vi "program_supply_arduino.vi"() -> ()   [LabVIEW 2018]
uses:
  <vilib>/MakerHub/LINX/Public/Peripherals/Analog/Analog Read 1 Chan.vi
  <vilib>/MakerHub/LINX/Public/Peripherals/PWM/PWM Set Duty Cycle 1 Chan.vi
  <vilib>/MakerHub/LINX/Public/Peripherals/Analog/Analog Read N Chans.vi
  <vilib>/MakerHub/LINX/Private/Local IO/LinxAnalogRead.vi
  <vilib>/MakerHub/LINX/Public/Utilities/Check Channel.vi
  <vilib>/MakerHub/LINX/Public/Utilities/Open Serial.vi
  <vilib>/MakerHub/LINX/Private/Utilties/Generate Error.vi
  <vilib>/MakerHub/LINX/Public/Peripherals/PWM/PWM Set Duty Cycle N Chans.vi
  <vilib>/MakerHub/LINX/LMH-LINX.lvlib
panel:
  in  "File Path":path
  in  "File Name":string
  out "通道六采集信号":dbl
  out "通道五采集信号":dbl
  out "通道四采集信号":dbl
  out "通道三采集信号":dbl
  in  "通道六（V）":dbl
  in  "通道五（V）":dbl
  in  "通道四（V）":dbl
  in  "通道三（V）":dbl
  out "通道二采集信号":dbl
  in  "通道二（V）":dbl
  in  "?":string
  out "通道一采集信号":dbl
  in  "停止":bool
  in  "通道一（V）":dbl
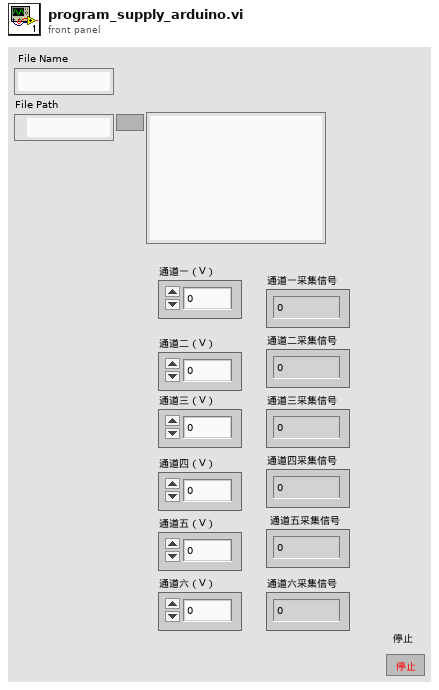
[diagram p1: front panel]
types:
  T1 = enum16{"open", "replace", "create", "open or create", "replace or create", "replace or create with confirmation"}
  T2 = typedef "LMH-LINX.lvlib/LINX Ref.ctl" = cluster{"IO":T3, "Interface":T4, "LINX Device Config":T5}
  T3 = typedef "LMH-LINX.lvlib/Platform.ctl" = enum16{"Remote", "Local"}
  T4 = typedef "LMH-LINX.lvlib/Interface.ctl" = enum16{"Serial", "TCP"}
  T5 = typedef "LMH-LINX.lvlib/Device.lvlib/LINX Device Config.ctl" = cluster{"Interface":T4, "COM Port":refnum<visa-resource-name>, "TCP Configuration":T6, "Device Family":u8, "Device ID":u8, "Device Name":string, "TCP Ref":refnum<k5>, "Channels":T7}
  T6 = typedef "LMH-LINX.lvlib/Device.lvlib/TCP Config.ctl" = cluster{"IP Address":string, "Port":u16}
  T7 = typedef "LMH-LINX.lvlib/Channels.ctl" = cluster{"DI":u8[], "DO":u8[], "AI":u8[], "AO":u8[], "PWM":u8[], "QE":u8[], "UART":u8[], "I2C 2":u8[], "SPI":u8[], "CAN":u8[], "Servo":u8[], "AI Ref (V)":dbl, "AI Resolution (Bits)":u8, "AO Ref (V)":dbl, "AO Resolution (Bits)":u8}
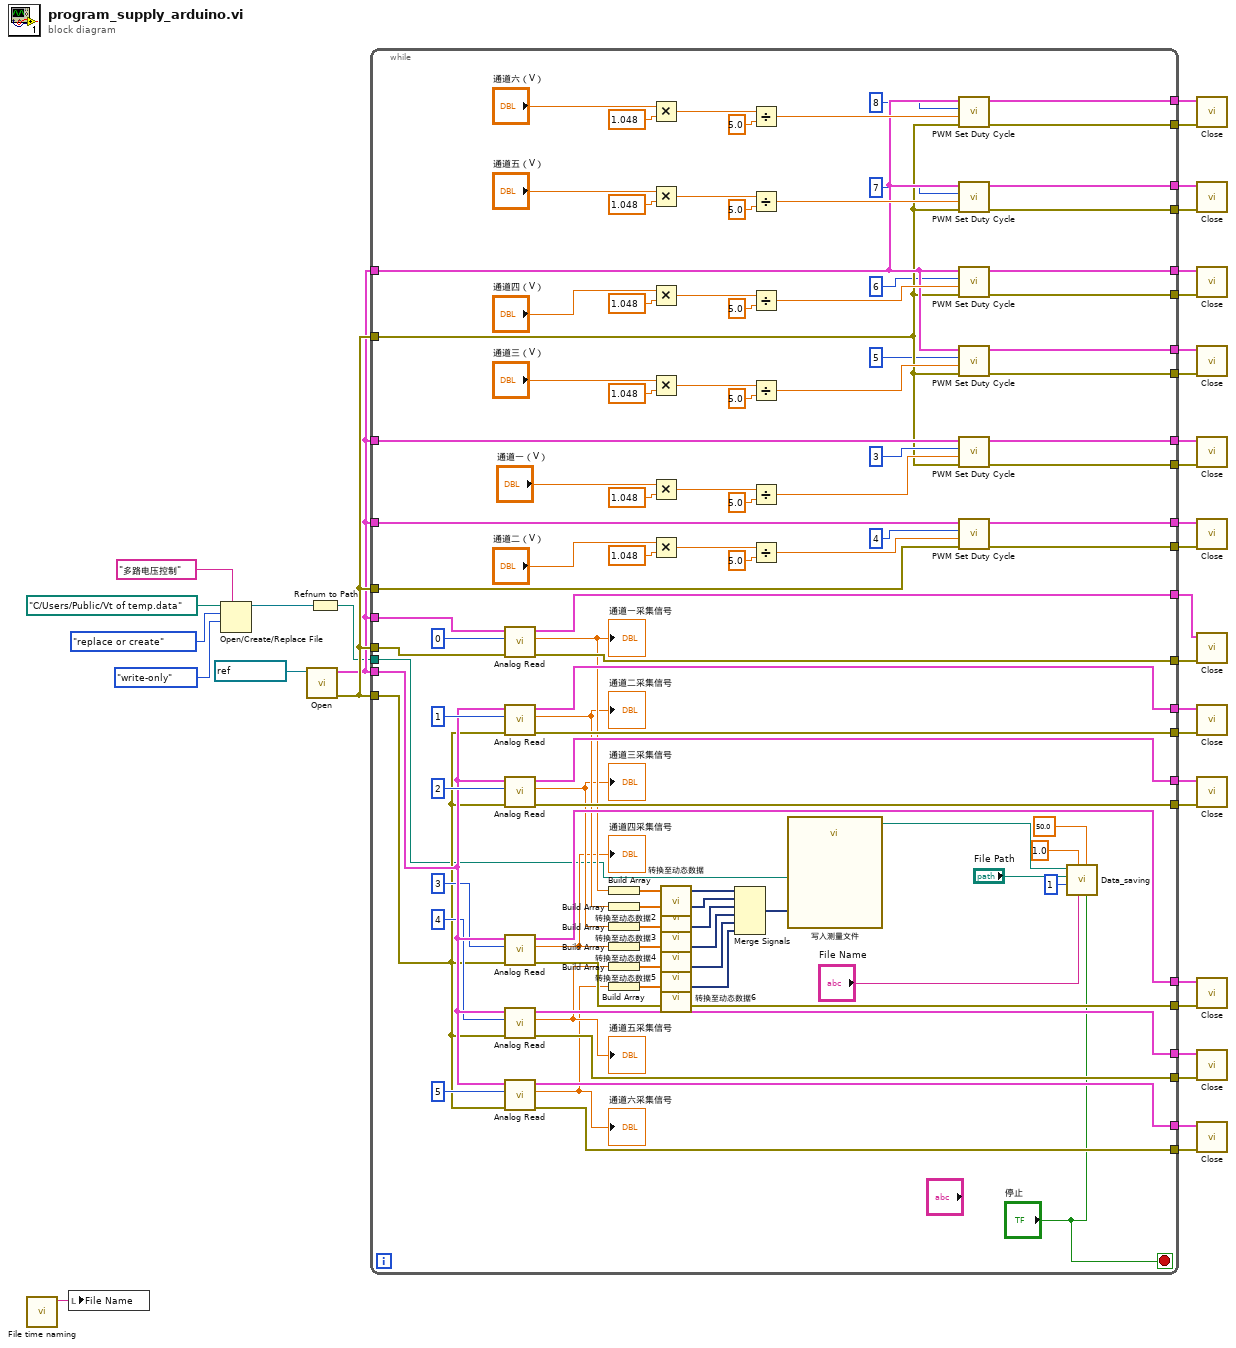
[diagram p0: block diagram]
diagram:
  n1 = call "File time naming.vi"() -> ("result string"=w1:string)  [unwired: 11 in]
  n2 = local write "File Name"(w1) -> ()
  n3 = Open/Create/Replace File(file path (use dialog)=path "C:/Users/Public/Vt of temp.data" ("文件路径（使用对话框）"), prompt="多路电压控制" ("提示"), operation (0:open)=T1."replace or create" ("操作(0:open)"), access (0:read/write)=enum16{"read/write", "read-only", "write-only"}."write-only" ("权限(0:read/write)")) -> (refnum out=w4:refnum<file>)  [unwired: 2 in, 2 out]
  n4 = call-poly <vilib>:"Open.vi"("Serial Port"=refnum<visa-resource-name> "COM26") -> ("Error Out"=w27:errorcluster, "LINX Resource"=w24:T2)  [unwired: 8 in, 1 out]
  n5 = Refnum to Path(1:w4) -> (0:w3:path)
  n6 = while {
    tunnel: w24 -> [w136]
    tunnel: w27 -> [w88]
    tunnel: [w135] -> w33
    tunnel: [w134] -> w32
    tunnel: w24 -> [w133]
    tunnel: w27 -> [w132]
    tunnel: [w124] -> w31
    tunnel: [w123] -> w30
    tunnel: w24 -> [w122]
    tunnel: w27 -> [w121]
    tunnel: [w119] -> w29
    tunnel: [w118] -> w28
    tunnel: w24 -> [w74]
    tunnel: w27 -> [w70]
    tunnel: [w112] -> w26
    tunnel: [w111] -> w25
    tunnel: w24 -> [w89]
    tunnel: [w83] -> w23
    tunnel: [w82] -> w22
    tunnel: [w81] -> w21
    tunnel: [w80] -> w20
    tunnel: [w79] -> w19
    tunnel: [w78] -> w18
    tunnel: [w77] -> w17
    tunnel: [w76] -> w16
    tunnel: [w69] -> w15
    tunnel: [w68] -> w14
    tunnel: [w67] -> w13
    tunnel: [w66] -> w12
    tunnel: [w65] -> w11
    tunnel: [w64] -> w10
    tunnel: [w63] -> w9
    tunnel: [w62] -> w8
    tunnel: w3 -> [w39]
    stop <- "停止" stop-if-true
    n7 = call-poly <vilib>:"Analog Read.vi"("Error In"=w132, "Analog Channel"=u8 0, "LINX Resource"=w133) -> ("Error Out"=w124:errorcluster, "Voltage"=w57:dbl, "LINX Resource"=w123:T2)  [unwired: 5 in, 1 out]
    "通道一采集信号" <- w57
    n8 = call-poly <vilib>:"Analog Read.vi"("Error In"=w70, "Analog Channel"=u8 1, "LINX Resource"=w74) -> ("Error Out"=w111:errorcluster, "Voltage"=w51:dbl, "LINX Resource"=w112:T2)  [unwired: 5 in, 1 out]
    "通道二采集信号" <- w51
    n9 = call-poly <vilib>:"Analog Read.vi"("Error In"=w70, "Analog Channel"=u8 2, "LINX Resource"=w74) -> ("Error Out"=w62:errorcluster, "Voltage"=w50:dbl, "LINX Resource"=w63:T2)  [unwired: 5 in, 1 out]
    "通道三采集信号" <- w50
    n10 = call-poly <vilib>:"Analog Read.vi"("Error In"=w70, "Analog Channel"=u8 3, "LINX Resource"=w74) -> ("Error Out"=w64:errorcluster, "Voltage"=w49:dbl, "LINX Resource"=w65:T2)  [unwired: 5 in, 1 out]
    "通道四采集信号" <- w49
    n11 = call-poly <vilib>:"Analog Read.vi"("Error In"=w70, "Analog Channel"=u8 4, "LINX Resource"=w74) -> ("Error Out"=w66:errorcluster, "Voltage"=w48:dbl, "LINX Resource"=w67:T2)  [unwired: 5 in, 1 out]
    "通道五采集信号" <- w48
    n12 = call-poly <vilib>:"Analog Read.vi"("Error In"=w70, "Analog Channel"=u8 5, "LINX Resource"=w74) -> ("Error Out"=w68:errorcluster, "Voltage"=w47:dbl, "LINX Resource"=w69:T2)  [unwired: 5 in, 1 out]
    "通道六采集信号" <- w47
    n13 = Build Array(w57) -> (w58:dbl[])
    n14 = Build Array(w51) -> (w56:dbl[])
    n15 = Build Array(w50) -> (w55:dbl[])
    n16 = Build Array(w49) -> (w54:dbl[])
    n17 = Build Array(w48) -> (w53:dbl[])
    n18 = Build Array(w47) -> (w52:dbl[])
    n19 = Multiply(x="通道六（V）", y=1.048) -> (x*y=w94:dbl)
    n20 = Multiply(x="通道五（V）", y=1.048) -> (x*y=w98:dbl)
    n21 = Multiply(x="通道四（V）", y=1.048) -> (x*y=w102:dbl)
    n22 = Multiply(x="通道三（V）", y=1.048) -> (x*y=w106:dbl)
    n23 = Multiply(x="通道一（V）", y=1.048) -> (x*y=w127:dbl)
    n24 = Multiply(x="通道二（V）", y=1.048) -> (x*y=w114:dbl)
    n25 = call "转换至动态数据"("Array"=w58) -> ("Dynamic Data Type"=w46:dynamicdata)  [unwired: 3 in]
    n26 = call "转换至动态数据2"("Array"=w56) -> ("Dynamic Data Type"=w45:dynamicdata)  [unwired: 3 in]
    n27 = call "转换至动态数据3"("Array"=w55) -> ("Dynamic Data Type"=w44:dynamicdata)  [unwired: 3 in]
    n28 = call "转换至动态数据4"("Array"=w54) -> ("Dynamic Data Type"=w43:dynamicdata)  [unwired: 3 in]
    n29 = call "转换至动态数据5"("Array"=w53) -> ("Dynamic Data Type"=w42:dynamicdata)  [unwired: 3 in]
    n30 = call "转换至动态数据6"("Array"=w52) -> ("Dynamic Data Type"=w41:dynamicdata)  [unwired: 3 in]
    n31 = Merge Signals(w46, w45, w44, w43, w42, w41) -> (w40:dynamicdata)
    n32 = Divide(x=w94, y=5.0) -> (x/y=w90:dbl)
    n33 = Divide(x=w98, y=5.0) -> (x/y=w91:dbl)
    n34 = Divide(x=w102, y=5.0) -> (x/y=w92:dbl)
    n35 = Divide(x=w106, y=5.0) -> (x/y=w93:dbl)
    n36 = Divide(x=w127, y=5.0) -> (x/y=w126:dbl)
    n37 = Divide(x=w114, y=5.0) -> (x/y=w113:dbl)
    n38 = call "写入测量文件"("Signals"=w40, "Filename"=w39) -> ("Filename Out"=w38:path)  [unwired: 15 in, 2 out]
    n39 = call-poly <vilib>:"PWM Set Duty Cycle.vi"("Error In"=w88, "Duty Cycle (0-1)"=w90, "PWM Channel"=u8 8, "LINX Resource"=w89) -> ("Error Out"=w76:errorcluster, "LINX Resource"=w77:T2)  [unwired: 6 in]
    n40 = call-poly <vilib>:"PWM Set Duty Cycle.vi"("Error In"=w88, "Duty Cycle (0-1)"=w91, "PWM Channel"=u8 7, "LINX Resource"=w89) -> ("Error Out"=w78:errorcluster, "LINX Resource"=w79:T2)  [unwired: 6 in]
    n41 = call-poly <vilib>:"PWM Set Duty Cycle.vi"("Error In"=w88, "Duty Cycle (0-1)"=w92, "PWM Channel"=u8 6, "LINX Resource"=w89) -> ("Error Out"=w80:errorcluster, "LINX Resource"=w81:T2)  [unwired: 6 in]
    n42 = call-poly <vilib>:"PWM Set Duty Cycle.vi"("Error In"=w88, "Duty Cycle (0-1)"=w93, "PWM Channel"=u8 5, "LINX Resource"=w89) -> ("Error Out"=w82:errorcluster, "LINX Resource"=w83:T2)  [unwired: 6 in]
    n43 = call-poly <vilib>:"PWM Set Duty Cycle.vi"("Error In"=w88, "Duty Cycle (0-1)"=w126, "PWM Channel"=u8 3, "LINX Resource"=w136) -> ("Error Out"=w135:errorcluster, "LINX Resource"=w134:T2)  [unwired: 6 in]
    n44 = call-poly <vilib>:"PWM Set Duty Cycle.vi"("Error In"=w121, "Duty Cycle (0-1)"=w113, "PWM Channel"=u8 4, "LINX Resource"=w122) -> ("Error Out"=w118:errorcluster, "LINX Resource"=w119:T2)  [unwired: 6 in]
    n45 = call "Data_saving.vi"("Boolean"="停止", "Sampling Rate"=50.0, "File Name"="File Name", "Voltage Sensitivity\n1000 will be 1000"=1.0 ("Voltage Sensitivity\n1000 will be 1000"), "Number of Samples Per Channel"=1, "File Path"="File Path", "File name source"=w38) -> ()  [unwired: 5 in]
  }
  n46 = call <vilib>:"Close.vi"("Error In"=w16, "LINX Resource"=w17) -> ()  [unwired: 9 in, 1 out]
  n47 = call <vilib>:"Close.vi"("Error In"=w18, "LINX Resource"=w19) -> ()  [unwired: 9 in, 1 out]
  n48 = call <vilib>:"Close.vi"("Error In"=w20, "LINX Resource"=w21) -> ()  [unwired: 9 in, 1 out]
  n49 = call <vilib>:"Close.vi"("Error In"=w22, "LINX Resource"=w23) -> ()  [unwired: 9 in, 1 out]
  n50 = call <vilib>:"Close.vi"("Error In"=w33, "LINX Resource"=w32) -> ()  [unwired: 9 in, 1 out]
  n51 = call <vilib>:"Close.vi"("Error In"=w28, "LINX Resource"=w29) -> ()  [unwired: 9 in, 1 out]
  n52 = call <vilib>:"Close.vi"("Error In"=w31, "LINX Resource"=w30) -> ()  [unwired: 9 in, 1 out]
  n53 = call <vilib>:"Close.vi"("Error In"=w25, "LINX Resource"=w26) -> ()  [unwired: 9 in, 1 out]
  n54 = call <vilib>:"Close.vi"("Error In"=w8, "LINX Resource"=w9) -> ()  [unwired: 9 in, 1 out]
  n55 = call <vilib>:"Close.vi"("Error In"=w10, "LINX Resource"=w11) -> ()  [unwired: 9 in, 1 out]
  n56 = call <vilib>:"Close.vi"("Error In"=w12, "LINX Resource"=w13) -> ()  [unwired: 9 in, 1 out]
  n57 = call <vilib>:"Close.vi"("Error In"=w14, "LINX Resource"=w15) -> ()  [unwired: 9 in, 1 out]
